vi "FindAllInboundGObjects.vi"(8 "error in (no error)":errorcluster, 10 "Coordinates":T1, 11 "List of GObjects":refnum<vi>[](array[refnum])) -> (0 "error out":errorcluster, 1 "Inbound objects found?":bool, 2 "Outbound GObjects":refnum<vi>[](array[refnum]), 3 "Inbound GObjects":refnum<vi>[](array[refnum]))   [LabVIEW 2012]
doc: "Filters the input list of GObjects to return only those that contain the coordinate specified."
uses:
  <vilib>/Utility/miscctls.llb/LVPoint32TypeDef.ctl
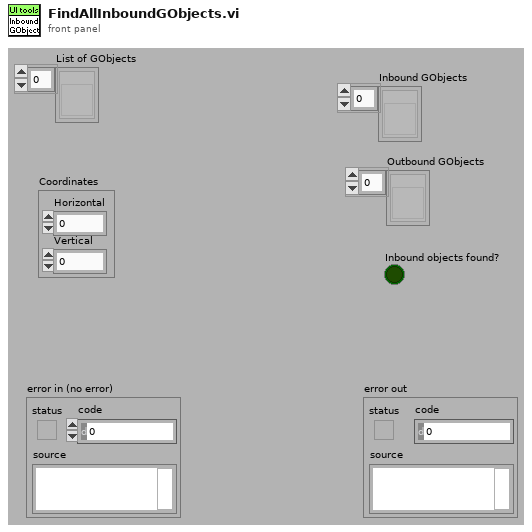
[diagram p1: front panel]
types:
  T1 = typedef "LVPoint32TypeDef.ctl" = cluster{"Horizontal":i32, "Vertical":i32}
  T2 = cluster{"left":i16, "top":i16, "right":i16, "bottom":i16}
  T3 = typedef "LVPositionTypeDef.ctl" = cluster{"Left":i32, "Top":i32}
  T4 = typedef "LVBoundsTypeDef.ctl" = cluster{"Width":u32, "Height":u32}
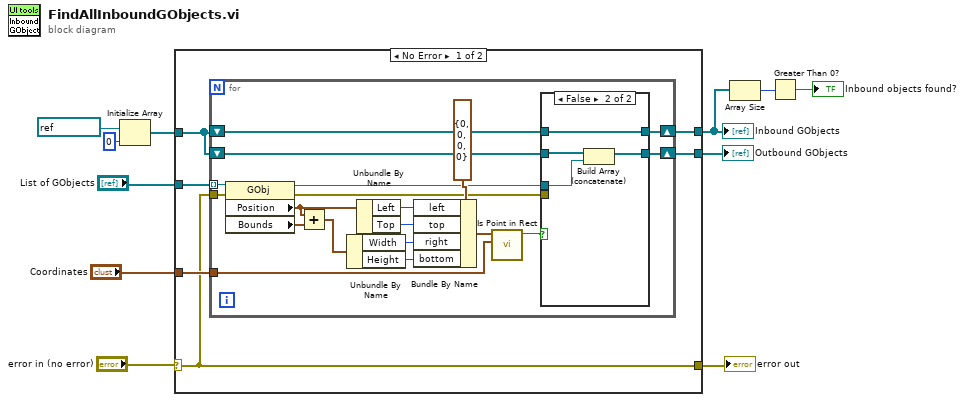
[diagram p0: block diagram]
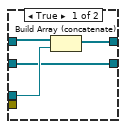
[diagram p2: hidden frame]
diagram:
  n1 = Initialize Array(refnum<vi> refnum ("GObject"), 0 ("dimension size")) -> (w5:refnum<vi>[])
  n2 = case shown="No Error" "error in (no error)" {
    selector: "error in (no error)" -> [w15 w47]
    tunnel: "List of GObjects" -> [w17 w46]
    tunnel: "Coordinates" -> [w16 _]
    tunnel: [w15 w47] -> w9
    tunnel: [w14 w45] -> w3
    tunnel: [w12 w46] -> w7
    tunnel: w5 -> [w13 w45]
    frame No Error {
      n3 = for {
        tunnel: w17 -> [w36] mode=indexing
        tunnel: w16 -> [w31]
        tunnel: w15 -> [w35]
        shift-right: [w19] -> w14
        shift-left: w13 -> [w21]
        shift-right: [w18] -> w12
        shift-left: w13 -> [w20]
        n4 = property class="GObj"(reference=w36, error in=w35) -> (reference out=w23:refnum<vi>, error out=w22:errorcluster, "Position"=w30:T3, "Bounds"=w34:T4)
        n5 = Add(x=w30, y=w34) -> (x+y=w27:T4)
        n6 = Unbundle By Name(w27) -> ("Width"=w26:u32, "Height"=w25:u32)
        n7 = Unbundle By Name(w30) -> ("Left"=w29:i32, "Top"=w28:i32)
        n8 = Bundle By Name(cluster=T2 {"left"=0, "top"=0, "right"=0, "bottom"=0} ("rect"), "left"=w29, "top"=w28, "right"=w26, "bottom"=w25) -> (w32:T2)
        n9 = call "Is Point in Rect.vi"("point"=w31, "rect"=w32) -> ("Point in Rect?"=w24:bool)  [unwired: 9 out]
        n10 = case shown="False" w24 {
          tunnel: w23 -> [w39 w44]
          tunnel: w22 -> [_ _]
          tunnel: w21 -> [w40 w41]
          tunnel: w20 -> [w37 w43]
          tunnel: [w38 w41] -> w19
          tunnel: [w37 w42] -> w18
          frame True {
            n11 = Build Array (concatenate)(w40, w39) -> (w38:refnum<vi>[])
          }
          frame False {
            n12 = Build Array (concatenate)(w43, w44) -> (w42:refnum<vi>[])
          }
        }
      }
    }
    frame Error {
    }
  }
  "error out" <- w9
  "Inbound GObjects" <- w3
  "Outbound GObjects" <- w7
  n13 = Array Size(array=w3) -> (size(s)=w2:i32)
  n14 = Greater Than 0?(x=w2) -> (x > 0?=→"Inbound objects found?":bool)
